vi "VISJS Viewer.vi"(4 "Extra Scripts":string, 5 "FileDependency In":map{path, T1}(c390), 6 "Options":string, 7 "OpenWebBrowser(False)":bool, 8 "error in":errorcluster, 9 "Embedd VISJS Librarya in HTMl File(False)":bool, 10 "HTMLFilePath":path, 11 "LibraryDependency":map{path, T3}(c390)) -> (0 "error out":errorcluster, 3 "HTMLFileContent":string)   [LabVIEW 2020, in "VISJS Viewer.lvlib"] (continued)
t}},{key:\"getPosition\",value:function(g){if(null==g)throw new TypeError(\"No id was specified for getPosition method.\");if(null==this.body.nodes[g])throw new ReferenceError(\"NodeId provided for getPosition does not exist. Provided: \".concat(g));return{x:Math.round(this.body.nodes[g].x),y:Math.round(this.body.nodes[g].y)}}},{key:\"storePositions\",value:function(){var g,t=[],A=this.body.data.nodes.getDataSet(),e=LN(A.get());try{for(e.s();!(g=e.n()).done;){var C=g.value,I=C.id,i=this.body.nodes[I],o=Math.round(i.x),n=Math.round(i.y);C.x===o&&C.y===n||t.push({id:I,x:o,y:n})}}catch(g){e.e(g)}finally{e.f()}A.update(t)}},{key:\"getBoundingBox\",value:function(g){if(void 0!==this.body.nodes[g])return this.body.nodes[g].shape.boundingBox}},{key:\"getConnectedNodes\",value:function(g,t){var A=[];if(void 0!==this.body.nodes[g])for(var e=this.body.nodes[g],C={},I=0;I<e.edges.length;I++){var i=e.edges[I];\"to\"!==t&&i.toId==e.id?void 0===C[i.fromId]&&(A.push(i.fromId),C[i.fromId]=!0):\"from\"!==t&&i.fromId==e.id&&void 0===C[i.toId]&&(A.push(i.toId),C[i.toId]=!0)}return A}},{key:\"getConnectedEdges\",value:function(g){var t=[];if(void 0!==this.body.nodes[g])for(var A=this.body.nodes[g],e=0;e<A.edges.length;e++)t.push(A.edges[e].id);else console.error(\"NodeId provided for getConnectedEdges does not exist. Provided: \",g);return t}},{key:\"moveNode\",value:function(g,t,A){var e=this;void 0!==this.body.nodes[g]?(this.body.nodes[g].x=Number(t),this.body.nodes[g].y=Number(A),wu((function(){e.body.emitter.emit(\"startSimulation\")}),0)):console.error(\"Node id supplied to moveNode does not exist. Provided: \",g)}}]),g}(),WN=qg,QN=P,UN=gg,_N=AA,KN=function(g){return void 0!==g&&(WN(g,\"value\")||WN(g,\"writable\"))},HN=T,XN=EI;TA({target:\"Reflect\",stat:!0},{get:function g(t,A){var e,C,I=arguments.length<3?t:arguments[2];return _N(t)===I?t[A]:(e=HN.f(t,A))?KN(e)?e.value:void 0===e.get?void 0:QN(e.get,I):UN(C=XN(t))?g(C,A,I):void 0}});var JN=A(tg.Reflect.get),qN=A(YT);function $N(){var g;\"undefined\"!=typeof Reflect&&JN?$N=Ab(g=JN).call(g):$N=function(g,t,A){var e=function(g,t){for(;!Object.prototype.hasOwnProperty.call(g,t)&&null!==(g=nb(g)););return g}(g,t);if(e){var C=qN(e,t);return C.get?C.get.call(arguments.length<3?g:A):C.value}};return $N.apply(this,arguments)}var gR=TA,tR=Math.hypot,AR=Math.abs,eR=Math.sqrt;gR({target:\"Math\",stat:!0,arity:2,forced:!!tR&&tR(1/0,NaN)!==1/0},{hypot:function(g,t){for(var A,e,C=0,I=0,i=arguments.length,o=0;I<i;)o<(A=AR(arguments[I++]))?(C=C*(e=o/A)*e+1,o=A):C+=A>0?(e=A/o)*e:A;return o===1/0?1/0:o*eR(C)}});var CR=A(tg.Math.hypot);function IR(g){var t=function(){if(\"undefined\"==typeof Reflect||!MT)return!1;if(MT.sham)return!1;if(\"function\"==typeof Proxy)return!0;try{return Boolean.prototype.valueOf.call(MT(Boolean,[],(function(){}))),!0}catch(g){return!1}}();return function(){var A,e=nb(g);if(t){var C=nb(this).constructor;A=MT(e,arguments,C)}else A=e.apply(this,arguments);return Ib(this,A)}}var iR=function(){function g(){cn(this,g)}return kd(g,null,[{key:\"transform\",value:function(g,t){Rh(g)||(g=[g]);for(var A=t.point.x,e=t.point.y,C=t.angle,I=t.length,i=0;i<g.length;++i){var o=g[i],n=o.x*Math.cos(C)-o.y*Math.sin(C),r=o.x*Math.sin(C)+o.y*Math.cos(C);o.x=A+I*n,o.y=e+I*r}}},{key:\"drawPath\",value:function(g,t){g.beginPath(),g.moveTo(t[0].x,t[0].y);for(var A=1;A<t.length;++A)g.lineTo(t[A].x,t[A].y);g.closePath()}}]),g}(),oR=function(g){Cb(A,g);var t=IR(A);function A(){return cn(this,A),t.apply(this,arguments)}return kd(A,null,[{key:\"draw\",value:function(g,t){if(t.image){g.save(),g.translate(t.point.x,t.point.y),g.rotate(Math.PI/2+t.angle);var A=null!=t.imageWidth?t.imageWidth:t.image.width,e=null!=t.imageHeight?t.imageHeight:t.image.height;t.image.drawImageAtPosition(g,1,-A/2,0,A,e),g.restore()}return!1}}]),A}(iR),nR=function(g){Cb(A,g);var t=IR(A);function A(){return cn(this,A),t.apply(this,arguments)}return kd(A,null,[{key:\"draw\",value:function(g,t){var A=[{x:0,y:0},{x:-1,y:.3},{x:-.9,y:0},{x:-1,y:-.3}];return iR.transform(A,t),iR.drawPath(g,A),!0}}]),A}(iR),rR=function(){function g(){cn(this,g)}return kd(g,null,[{key:\"draw\",value:function(g,t){var A=[{x:-1,y:0},{x:0,y:.3},{x:-.4,y:0},{x:0,y:-.3}];return iR.transform(A,t),iR.drawPath(g,A),!0}}]),g}(),sR=function(){function g(){cn(this,g)}return kd(g,null,[{key:\"draw\",value:function(g,t){var A={x:-.4,y:0};iR.transform(A,t),g.strokeStyle=g.fillStyle,g.fillStyle=\"rgba(0, 0, 0, 0)\";var e=Math.PI,C=t.angle-e/2,I=t.angle+e/2;return g.beginPath(),g.arc(A.x,A.y,.4*t.length,C,I,!1),g.stroke(),!0}}]),g}(),aR=function(){function g(){cn(this,g)}return kd(g,null,[{key:\"draw\",value:function(g,t){var A={x:-.3,y:0};iR.transform(A,t),g.strokeStyle=g.fillStyle,g.fillStyle=\"rgba(0, 0, 0, 0)\";var e=Math.PI,C=t.angle+e/2,I=t.angle+3*e/2;return g.beginPath(),g.arc(A.x,A.y,.4*t.length,C,I,!1),g.stroke(),!0}}]),g}(),dR=function(){function g(){cn(this,g)}return kd(g,null,[{key:\"draw\",value:function(g,t){var A=[{x:.02,y:0},{x:-1,y:.3},{x:-1,y:-.3}];return iR.transform(A,t),iR.drawPath(g,A),!0}}]),g}(),hR=function(){function g(){cn(this,g)}return kd(g,null,[{key:\"draw\",value:function(g,t){var A=[{x:0,y:.3},{x:0,y:-.3},{x:-1,y:0}];return iR.transform(A,t),iR.drawPath(g,A),!0}}]),g}(),lR=function(){function g(){cn(this,g)}return kd(g,null,[{key:\"draw\",value:function(g,t){var A={x:-.4,y:0};return iR.transform(A,t),Le(g,A.x,A.y,.4*t.length),!0}}]),g}(),cR=function(){function g(){cn(this,g)}return kd(g,null,[{key:\"draw\",value:function(g,t){var A=[{x:0,y:.5},{x:0,y:-.5},{x:-.15,y:-.5},{x:-.15,y:.5}];return iR.transform(A,t),iR.drawPath(g,A),!0}}]),g}(),uR=function(){function g(){cn(this,g)}return kd(g,null,[{key:\"draw\",value:function(g,t){var A=[{x:0,y:.3},{x:0,y:-.3},{x:-.6,y:-.3},{x:-.6,y:.3}];return iR.transform(A,t),iR.drawPath(g,A),!0}}]),g}(),pR=function(){function g(){cn(this,g)}return kd(g,null,[{key:\"draw\",value:function(g,t){var A=[{x:0,y:0},{x:-.5,y:-.3},{x:-1,y:0},{x:-.5,y:.3}];return iR.transform(A,t),iR.drawPath(g,A),!0}}]),g}(),fR=function(){function g(){cn(this,g)}return kd(g,null,[{key:\"draw\",value:function(g,t){var A=[{x:-1,y:.3},{x:-.5,y:0},{x:-1,y:-.3},{x:0,y:0}];return iR.transform(A,t),iR.drawPath(g,A),!0}}]),g}(),vR=function(){function g(){cn(this,g)}return kd(g,null,[{key:\"draw\",value:function(g,t){var A;switch(t.type&&(A=t.type.toLowerCase()),A){case\"image\":return oR.draw(g,t);case\"circle\":return lR.draw(g,t);case\"box\":return uR.draw(g,t);case\"crow\":return rR.draw(g,t);case\"curve\":return sR.draw(g,t);case\"diamond\":return pR.draw(g,t);case\"inv_curve\":return aR.draw(g,t);case\"triangle\":return dR.draw(g,t);case\"inv_triangle\":return hR.draw(g,t);case\"bar\":return cR.draw(g,t);case\"vee\":return fR.draw(g,t);default:return nR.draw(g,t)}}}]),g}();function yR(g,t){var A=Lh(g);if(BT){var e=BT(g);t&&(e=pc(e).call(e,(function(t){return WT(g,t).enumerable}))),A.push.apply(A,e)}return A}function mR(g){for(var t=1;t<arguments.length;t++){var A,e,C=null!=arguments[t]?arguments[t]:{};t%2?Cl(A=yR(Object(C),!0)).call(A,(function(t){rb(g,t,C[t])})):HT?AD(g,HT(C)):Cl(e=yR(Object(C))).call(e,(function(t){fT(g,t,WT(C,t))}))}return g}var bR=function(){function g(t,A,e){cn(this,g),this._body=A,this._labelModule=e,this.color={},this.colorDirty=!0,this.hoverWidth=1.5,this.selectionWidth=2,this.setOptions(t),this.fromPoint=this.from,this.toPoint=this.to}return kd(g,[{key:\"connect\",value:function(){this.from=this._body.nodes[this.options.from],this.to=this._body.nodes[this.options.to]}},{key:\"cleanup\",value:function(){return!1}},{key:\"setOptions\",value:function(g){this.options=g,this.from=this._body.nodes[this.options.from],this.to=this._body.nodes[this.options.to],this.id=this.options.id}},{key:\"drawLine\",value:function(g,t,A,e){var C=arguments.length>4&&void 0!==arguments[4]?arguments[4]:this.getViaNode();g.strokeStyle=this.getColor(g,t),g.lineWidth=t.width,!1!==t.dashes?this._drawDashedLine(g,t,C):this._drawLine(g,t,C)}},{key:\"_drawLine\",value:function(g,t,A,e,C){if(this.from!=this.to)this._line(g,t,A,e,C);else{var I=lh(this._getCircleData(g),3),i=I[0],o=I[1],n=I[2];this._circle(g,t,i,o,n)}}},{key:\"_drawDashedLine\",value:function(g,t,A,e,C){g.lineCap=\"round\";var I=Rh(t.dashes)?t.dashes:[5,5];if(void 0!==g.setLineDash){if(g.save(),g.setLineDash(I),g.lineDashOffset=0,this.from!=this.to)this._line(g,t,A);else{var i=lh(this._getCircleData(g),3),o=i[0],n=i[1],r=i[2];this._circle(g,t,o,n,r)}g.setLineDash([0]),g.lineDashOffset=0,g.restore()}else{if(this.from!=this.to)Qe(g,this.from.x,this.from.y,this.to.x,this.to.y,I);else{var s=lh(this._getCircleData(g),3),a=s[0],d=s[1],h=s[2];this._circle(g,t,a,d,h)}this.enableShadow(g,t),g.stroke(),this.disableShadow(g,t)}}},{key:\"findBorderPosition\",value:function(g,t,A){return this.from!=this.to?this._findBorderPosition(g,t,A):this._findBorderPositionCircle(g,t,A)}},{key:\"findBorderPositions\",value:function(g){if(this.from!=this.to)return{from:this._findBorderPosition(this.from,g),to:this._findBorderPosition(this.to,g)};var t,A=lh(wh(t=this._getCircleData(g)).call(t,0,2),2),e=A[0],C=A[1];return{from:this._findBorderPositionCircle(this.from,g,{x:e,y:C,low:.25,high:.6,direction:-1}),to:this._findBorderPositionCircle(this.from,g,{x:e,y:C,low:.6,high:.8,direction:1})}}},{key:\"_getCircleData\",value:function(g){var t=this.options.selfReference.size;void 0!==g&&void 0===this.from.shape.width&&this.from.shape.resize(g);var A=UD(g,this.options.selfReference.angle,t,this.from);return[A.x,A.y,t]}},{key:\"_pointOnCircle\",value:function(g,t,A,e){var C=2*e*Math.PI;return{x:g+A*Math.cos(C),y:t-A*Math.sin(C)}}},{key:\"_findBorderPositionCircle\",value:function(g,t,A){var e,C=A.x,I=A.y,i=A.low,o=A.high,n=A.direction,r=this.options.selfReference.size,s=.5*(i+o),a=0;!0===this.options.arrowStrikethrough&&(-1===n?a=this.options.endPointOffset.from:1===n&&(a=this.options.endPointOffset.to));var d=0;do{s=.5*(i+o),e=this._pointOnCircle(C,I,r,s);var h=Math.atan2(g.y-e.y,g.x-e.x),l=g.distanceToBorder(t,h)+a-Math.sqrt(Math.pow(e.x-g.x,2)+Math.pow(e.y-g.y,2));if(Math.abs(l)<.05)break;l>0?n>0?i=s:o=s:n>0?o=s:i=s,++d}while(i<=o&&d<10);return mR(mR({},e),{},{t:s})}},{key:\"getLineWidth\",value:function(g,t){return!0===g?Math.max(this.selectionWidth,.3/this._body.view.scale):!0===t?Math.max(this.hoverWidth,.3/this._body.view.scale):Math.max(this.options.width,.3/this._body.view.scale)}},{key:\"getColor\",value:function(g,t){if(!1!==t.inheritsColor){if(\"both\"===t.inheritsColor&&this.from.id!==this.to.id){var A=g.createLinearGradient(this.from.x,this.from.y,this.to.x,this.to.y),e=this.from.options.color.highlight.border,C=this.to.options.color.highlight.border;return!1===this.from.selected&&!1===this.to.selected?(e=ev(this.from.options.color.border,t.opacity),C=ev(this.to.options.color.border,t.opacity)):!0===this.from.selected&&!1===this.to.selected?C=this.to.options.color.border:!1===this.from.selected&&!0===this.to.selected&&(e=this.from.options.color.border),A.addColorStop(0,e),A.addColorStop(1,C),A}return\"to\"===t.inheritsColor?ev(this.to.options.color.border,t.opacity):ev(this.from.options.color.border,t.opacity)}return ev(t.color,t.opacity)}},{key:\"_circle\",value:function(g,t,A,e,C){this.enableShadow(g,t);var I=0,i=2*Math.PI;if(!this.options.selfReference.renderBehindTheNode){var o=this.options.selfReference.angle,n=this.options.selfReference.angle+Math.PI,r=this._findBorderPositionCircle(this.from,g,{x:A,y:e,low:o,high:n,direction:-1}),s=this._findBorderPositionCircle(this.from,g,{x:A,y:e,low:o,high:n,direction:1});I=Math.atan2(r.y-e,r.x-A),i=Math.atan2(s.y-e,s.x-A)}g.beginPath(),g.arc(A,e,C,I,i,!1),g.stroke(),this.disableShadow(g,t)}},{key:\"getDistanceToEdge\",value:function(g,t,A,e,C,I){if(this.from!=this.to)return this._getDistanceToEdge(g,t,A,e,C,I);var i=lh(this._getCircleData(void 0),3),o=i[0],n=i[1],r=i[2],s=o-C,a=n-I;return Math.abs(Math.sqrt(s*s+a*a)-r)}},{key:\"_getDistanceToLine\",value:function(g,t,A,e,C,I){var i=A-g,o=e-t,n=((C-g)*i+(I-t)*o)/(i*i+o*o);n>1?n=1:n<0&&(n=0);var r=g+n*i-C,s=t+n*o-I;return Math.sqrt(r*r+s*s)}},{key:\"getArrowData\",value:function(g,t,A,e,C,I){var i,o,n,r,s,a,d,h=I.width;\"from\"===t?(n=this.from,r=this.to,s=I.fromArrowScale<0,a=Math.abs(I.fromArrowScale),d=I.fromArrowType):\"to\"===t?(n=this.to,r=this.from,s=I.toArrowScale<0,a=Math.abs(I.toArrowScale),d=I.toArrowType):(n=this.to,r=this.from,s=I.middleArrowScale<0,a=Math.abs(I.middleArrowScale),d=I.middleArrowType);var l=15*a+3*h;if(n!=r){var c=l/CR(n.x-r.x,n.y-r.y);if(\"middle\"!==t)if(!0===this.options.smooth.enabled){var u=this._findBorderPosition(n,g,{via:A}),p=this.getPoint(u.t+c*(\"from\"===t?1:-1),A);i=Math.atan2(u.y-p.y,u.x-p.x),o=u}else i=Math.atan2(n.y-r.y,n.x-r.x),o=this._findBorderPosition(n,g);else{var f=(s?-c:c)/2,v=this.getPoint(.5+f,A),y=this.getPoint(.5-f,A);i=Math.atan2(v.y-y.y,v.x-y.x),o=this.getPoint(.5,A)}}else{var m=lh(this._getCircleData(g),3),b=m[0],w=m[1],k=m[2];if(\"from\"===t){var x=this.options.selfReference.angle,E=this.options.selfReference.angle+Math.PI,O=this._findBorderPositionCircle(this.from,g,{x:b,y:w,low:x,high:E,direction:-1});i=-2*O.t*Math.PI+1.5*Math.PI+.1*Math.PI,o=O}else if(\"to\"===t){var T=this.options.selfReference.angle,D=this.options.selfReference.angle+Math.PI,N=this._findBorderPositionCircle(this.from,g,{x:b,y:w,low:T,high:D,direction:1});i=-2*N.t*Math.PI+1.5*Math.PI-1.1*Math.PI,o=N}else{var R=this.options.selfReference.angle/(2*Math.PI);o=this._pointOnCircle(b,w,k,R),i=-2*R*Math.PI+1.5*Math.PI+.1*Math.PI}}return{point:o,core:{x:o.x-.9*l*Math.cos(i),y:o.y-.9*l*Math.sin(i)},angle:i,length:l,type:d}}},{key:\"drawArrowHead\",value:function(g,t,A,e,C){g.strokeStyle=this.getColor(g,t),g.fillStyle=g.strokeStyle,g.lineWidth=t.width,vR.draw(g,C)&&(this.enableShadow(g,t),Bu(g).call(g),this.disableShadow(g,t))}},{key:\"enableShadow\",value:function(g,t){!0===t.shadow&&(g.shadowColor=t.shadowColor,g.shadowBlur=t.shadowSize,g.shadowOffsetX=t.shadowX,g.shadowOffsetY=t.shadowY)}},{key:\"disableShadow\",value:function(g,t){!0===t.shadow&&(g.shadowColor=\"rgba(0,0,0,0)\",g.shadowBlur=0,g.shadowOffsetX=0,g.shadowOffsetY=0)}},{key:\"drawBackground\",value:function(g,t){if(!1!==t.background){var A={strokeStyle:g.strokeStyle,lineWidth:g.lineWidth,dashes:g.dashes};g.strokeStyle=t.backgroundColor,g.lineWidth=t.backgroundSize,this.setStrokeDashed(g,t.backgroundDashes),g.stroke(),g.strokeStyle=A.strokeStyle,g.lineWidth=A.lineWidth,g.dashes=A.dashes,this.setStrokeDashed(g,t.dashes)}}},{key:\"setStrokeDashed\",value:function(g,t){if(!1!==t)if(void 0!==g.setLineDash){var A=Rh(t)?t:[5,5];g.setLineDash(A)}else console.warn(\"setLineDash is not supported in this browser. The dashed stroke cannot be used.\");else void 0!==g.setLineDash?g.setLineDash([]):console.warn(\"setLineDash is not supported in this browser. The dashed stroke cannot be used.\")}}]),g}();function wR(g,t){var A=Lh(g);if(BT){var e=BT(g);t&&(e=pc(e).call(e,(function(t){return WT(g,t).enumerable}))),A.push.apply(A,e)}return A}function kR(g){for(var t=1;t<arguments.length;t++){var A,e,C=null!=arguments[t]?arguments[t]:{};t%2?Cl(A=wR(Object(C),!0)).call(A,(function(t){rb(g,t,C[t])})):HT?AD(g,HT(C)):Cl(e=wR(Object(C))).call(e,(function(t){fT(g,t,WT(C,t))}))}return g}function xR(g){var t=function(){if(\"undefined\"==typeof Reflect||!MT)return!1;if(MT.sham)return!1;if(\"function\"==typeof Proxy)return!0;try{return Boolean.prototype.valueOf.call(MT(Boolean,[],(function(){}))),!0}catch(g){return!1}}();return function(){var A,e=nb(g);if(t){var C=nb(this).constructor;A=MT(e,arguments,C)}else A=e.apply(this,arguments);return Ib(this,A)}}var ER=function(g){Cb(A,g);var t=xR(A);function A(g,e,C){return cn(this,A),t.call(this,g,e,C)}return kd(A,[{key:\"_findBorderPositionBezier\",value:function(g,t){var A,e,C=arguments.length>2&&void 0!==arguments[2]?arguments[2]:this._getViaCoordinates(),I=!1,i=1,o=0,n=this.to,r=this.options.endPointOffset?this.options.endPointOffset.to:0;g.id===this.from.id&&(n=this.from,I=!0,r=this.options.endPointOffset?this.options.endPointOffset.from:0),!1===this.options.arrowStrikethrough&&(r=0);var s=0;do{e=.5*(o+i),A=this.getPoint(e,C);var a=Math.atan2(n.y-A.y,n.x-A.x),d=n.distanceToBorder(t,a)+r-Math.sqrt(Math.pow(A.x-n.x,2)+Math.pow(A.y-n.y,2));if(Math.abs(d)<.2)break;d<0?!1===I?o=e:i=e:!1===I?i=e:o=e,++s}while(o<=i&&s<10);return kR(kR({},A),{},{t:e})}},{key:\"_getDistanceToBezierEdge\",value:function(g,t,A,e,C,I,i){var o,n,r,s,a,d=1e9,h=g,l=t;for(n=1;n<10;n++)r=.1*n,s=Math.pow(1-r,2)*g+2*r*(1-r)*i.x+Math.pow(r,2)*A,a=Math.pow(1-r,2)*t+2*r*(1-r)*i.y+Math.pow(r,2)*e,n>0&&(d=(o=this._getDistanceToLine(h,l,s,a,C,I))<d?o:d),h=s,l=a;return d}},{key:\"_bezierCurve\",value:function(g,t,A,e){g.beginPath(),g.moveTo(this.fromPoint.x,this.fromPoint.y),null!=A&&null!=A.x?null!=e&&null!=e.x?g.bezierCurveTo(A.x,A.y,e.x,e.y,this.toPoint.x,this.toPoint.y):g.quadraticCurveTo(A.x,A.y,this.toPoint.x,this.toPoint.y):g.lineTo(this.toPoint.x,this.toPoint.y),this.drawBackground(g,t),this.enableShadow(g,t),g.stroke(),this.disableShadow(g,t)}},{key:\"getViaNode\",value:function(){return this._getViaCoordinates()}}]),A}(bR);function OR(g){var t=function(){if(\"undefined\"==typeof Reflect||!MT)return!1;if(MT.sham)return!1;if(\"function\"==typeof Proxy)return!0;try{return Boolean.prototype.valueOf.call(MT(Boolean,[],(function(){}))),!0}catch(g){return!1}}();return function(){var A,e=nb(g);if(t){var C=nb(this).constructor;A=MT(e,arguments,C)}else A=e.apply(this,arguments);return Ib(this,A)}}var TR=function(g){Cb(A,g);var t=OR(A);function A(g,e,C){var I;return cn(this,A),(I=t.call(this,g,e,C)).via=I.via,I._boundFunction=function(){I.positionBezierNode()},I._body.emitter.on(\"_repositionBezierNodes\",I._boundFunction),I}return kd(A,[{key:\"setOptions\",value:function(g){$N(nb(A.prototype),\"setOptions\",this).call(this,g);var t=!1;this.options.physics!==g.physics&&(t=!0),this.options=g,this.id=this.options.id,this.from=this._body.nodes[this.options.from],this.to=this._body.nodes[this.options.to],this.setupSupportNode(),this.connect(),!0===t&&(this.via.setOptions({physics:this.options.physics}),this.positionBezierNode())}},{key:\"connect\",value:function(){this.from=this._body.nodes[this.options.from],this.to=this._body.nodes[this.options.to],void 0===this.from||void 0===this.to||!1===this.options.physics||this.from.id===this.to.id?this.via.setOptions({physics:!1}):this.via.setOptions({physics:!0})}},{key:\"cleanup\",value:function(){return this._body.emitter.off(\"_repositionBezierNodes\",this._boundFunction),void 0!==this.via&&(delete this._body.nodes[this.via.id],this.via=void 0,!0)}},{key:\"setupSupportNode\",value:function(){if(void 0===this.via){var g=\"edgeId:\"+this.id,t=this._body.functions.createNode({id:g,shape:\"circle\",physics:!0,hidden:!0});this._body.nodes[g]=t,this.via=t,this.via.parentEdgeId=this.id,this.positionBezierNode()}}},{key:\"positionBezierNode\",value:function(){void 0!==this.via&&void 0!==this.from&&void 0!==this.to?(this.via.x=.5*(this.from.x+this.to.x),this.via.y=.5*(this.from.y+this.to.y)):void 0!==this.via&&(this.via.x=0,this.via.y=0)}},{key:\"_line\",value:function(g,t,A){this._bezierCurve(g,t,A)}},{key:\"_getViaCoordinates\",value:function(){return this.via}},{key:\"getViaNode\",value:function(){return this.via}},{key:\"getPoint\",value:function(g){var t=arguments.length>1&&void 0!==arguments[1]?arguments[1]:this.via;if(this.from===this.to){var A=lh(this._getCircleData(),3),e=A[0],C=A[1],I=A[2],i=2*Math.PI*(1-g);return{x:e+I*Math.sin(i),y:C+I-I*(1-Math.cos(i))}}return{x:Math.pow(1-g,2)*this.fromPoint.x+2*g*(1-g)*t.x+Math.pow(g,2)*this.toPoint.x,y:Math.pow(1-g,2)*this.fromPoint.y+2*g*(1-g)*t.y+Math.pow(g,2)*this.toPoint.y}}},{key:\"_findBorderPosition\",value:function(g,t){return this._findBorderPositionBezier(g,t,this.via)}},{key:\"_getDistanceToEdge\",value:function(g,t,A,e,C,I){return this._getDistanceToBezierEdge(g,t,A,e,C,I,this.via)}}]),A}(ER);function DR(g){var t=
